vi "Query System Capabilities.vi"(8 "error in (no error)":errorcluster, 11 "VISA resource name":refnum<visa-resource-name>) -> (0 "error out":errorcluster, 2 "Capabilities":string, 3 "VISA resource name out":refnum<visa-resource-name>)   [LabVIEW 2018, in "XP Power PLS600.lvlib"]
doc: "Displays the unit capability string."
uses:
  XP Power PLS600.lvlib
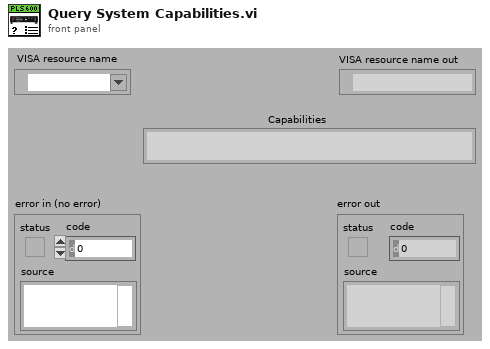
[diagram p1: front panel]
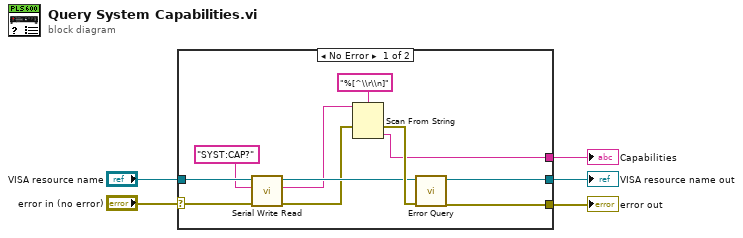
[diagram p0: block diagram]
diagram:
  n1 = case shown="No Error" "error in (no error)" {
    selector: "error in (no error)" -> [w7 w18]
    tunnel: [w16 w17] -> w5
    tunnel: [w15 w18] -> w4
    tunnel: "VISA resource name" -> [w12 w17]
    tunnel: [w6 _] -> w1
    frame No Error {
      n2 = call "Serial Write Read.vi"("error in (no error)"=w7, "Write Buffer"="SYST:CAP?", "VISA resource name"=w12) -> ("error out"=w8:errorcluster, "Read Buffer"=w9:string, "VISA resource name out"=w10:refnum<visa-resource-name>)  [unwired: 6 in]
      n3 = Scan From String(format string="%[^\\r\\n]", input string=w9, error in=w8) -> (error out=w13:errorcluster, output 1=w6:string)  [unwired: 2 in, 2 out]
      n4 = call "Error Query.vi"("error in (no error)"=w13, "VISA resource name"=w10) -> ("error out"=w15:errorcluster, "VISA resource name out"=w16:refnum<visa-resource-name>)  [unwired: 6 in, 2 out]
    }
    frame Error {
    }
  }
  "VISA resource name out" <- w5
  "error out" <- w4
  "Capabilities" <- w1
